vi "ShooterSpeed.vi"(8 "semaphore":T1, 9 "Bottom Shooter":T2, 10 "Top Shooter":T2) -> ()   [LabVIEW 2011]
uses:
  <vilib>/Rock Robotics/WPI/MotorControl/WPI_MotorControlDeviceRef.ctl
  <vilib>/Rock Robotics/SystemInterfaces/Typedef/FPGA_TypedefDigitalModule.ctl
  <vilib>/Rock Robotics/SystemInterfaces/DIO/FPGA_DIOPWMChannel.ctl
  <vilib>/Rock Robotics/WPI/PWM/WPI_PWMDeadband.ctl
  <vilib>/Rock Robotics/WPI/CAN/Jaguar/SubVIs/WPI_CANJaguar_ControlMode.ctl
  <vilib>/Rock Robotics/WPI/PWM/WPI_PWMTransform_ConPane.ctl
  Robot Global Data.vi
  <vilib>/addons/control/pid/NI_PID_pid.lvlib
panel:
  in  "t":dbl
  out "PID Out":dbl(graph)
  out "Error":dbl(graph)
  in  "Shooter Feed Forward":cluster{"Speed":sgl, "Setpoint":sgl}[](array[cluster])=[{"Speed"=0.0, "Setpoint"=0.0}, {"Speed"=1700.0, "Setpoint"=0.3}, {"Speed"=2300.0, "Setpoint"=0.4}, {"Speed"=3000.0, "Setpoint"=0.5}, {"Speed"=3600.0, "Setpoint"=0.6}, {"Speed"=4200.0, "Setpoint"=0.7}, {"Speed"=5000.0, "Setpoint"=0.8}, {"Speed"=6000.0, "Setpoint"=0.9}, {"Speed"=6400.0, "Setpoint"=1.0}]
  out "error out 2":errorcluster
  out "error out":errorcluster
  out "RPM":dbl(graph)
  in  "PID gains":T8={"proportional gain (Kc)"=8.0, "integral time (Ti, min)"=0.01, "derivative time (Td, min)"=0.0} {"derivative time (Td, min)" format="%.3f"; "integral time (Ti, min)" format="%.3f"; "proportional gain (Kc)" format="%.3f"}
  in  "output range":cluster{"output high":dbl, "output low":dbl}={"output high"=0.5, "output low"=-0.5} {"output low" format="%.2f"; "output high" format="%.2f"}
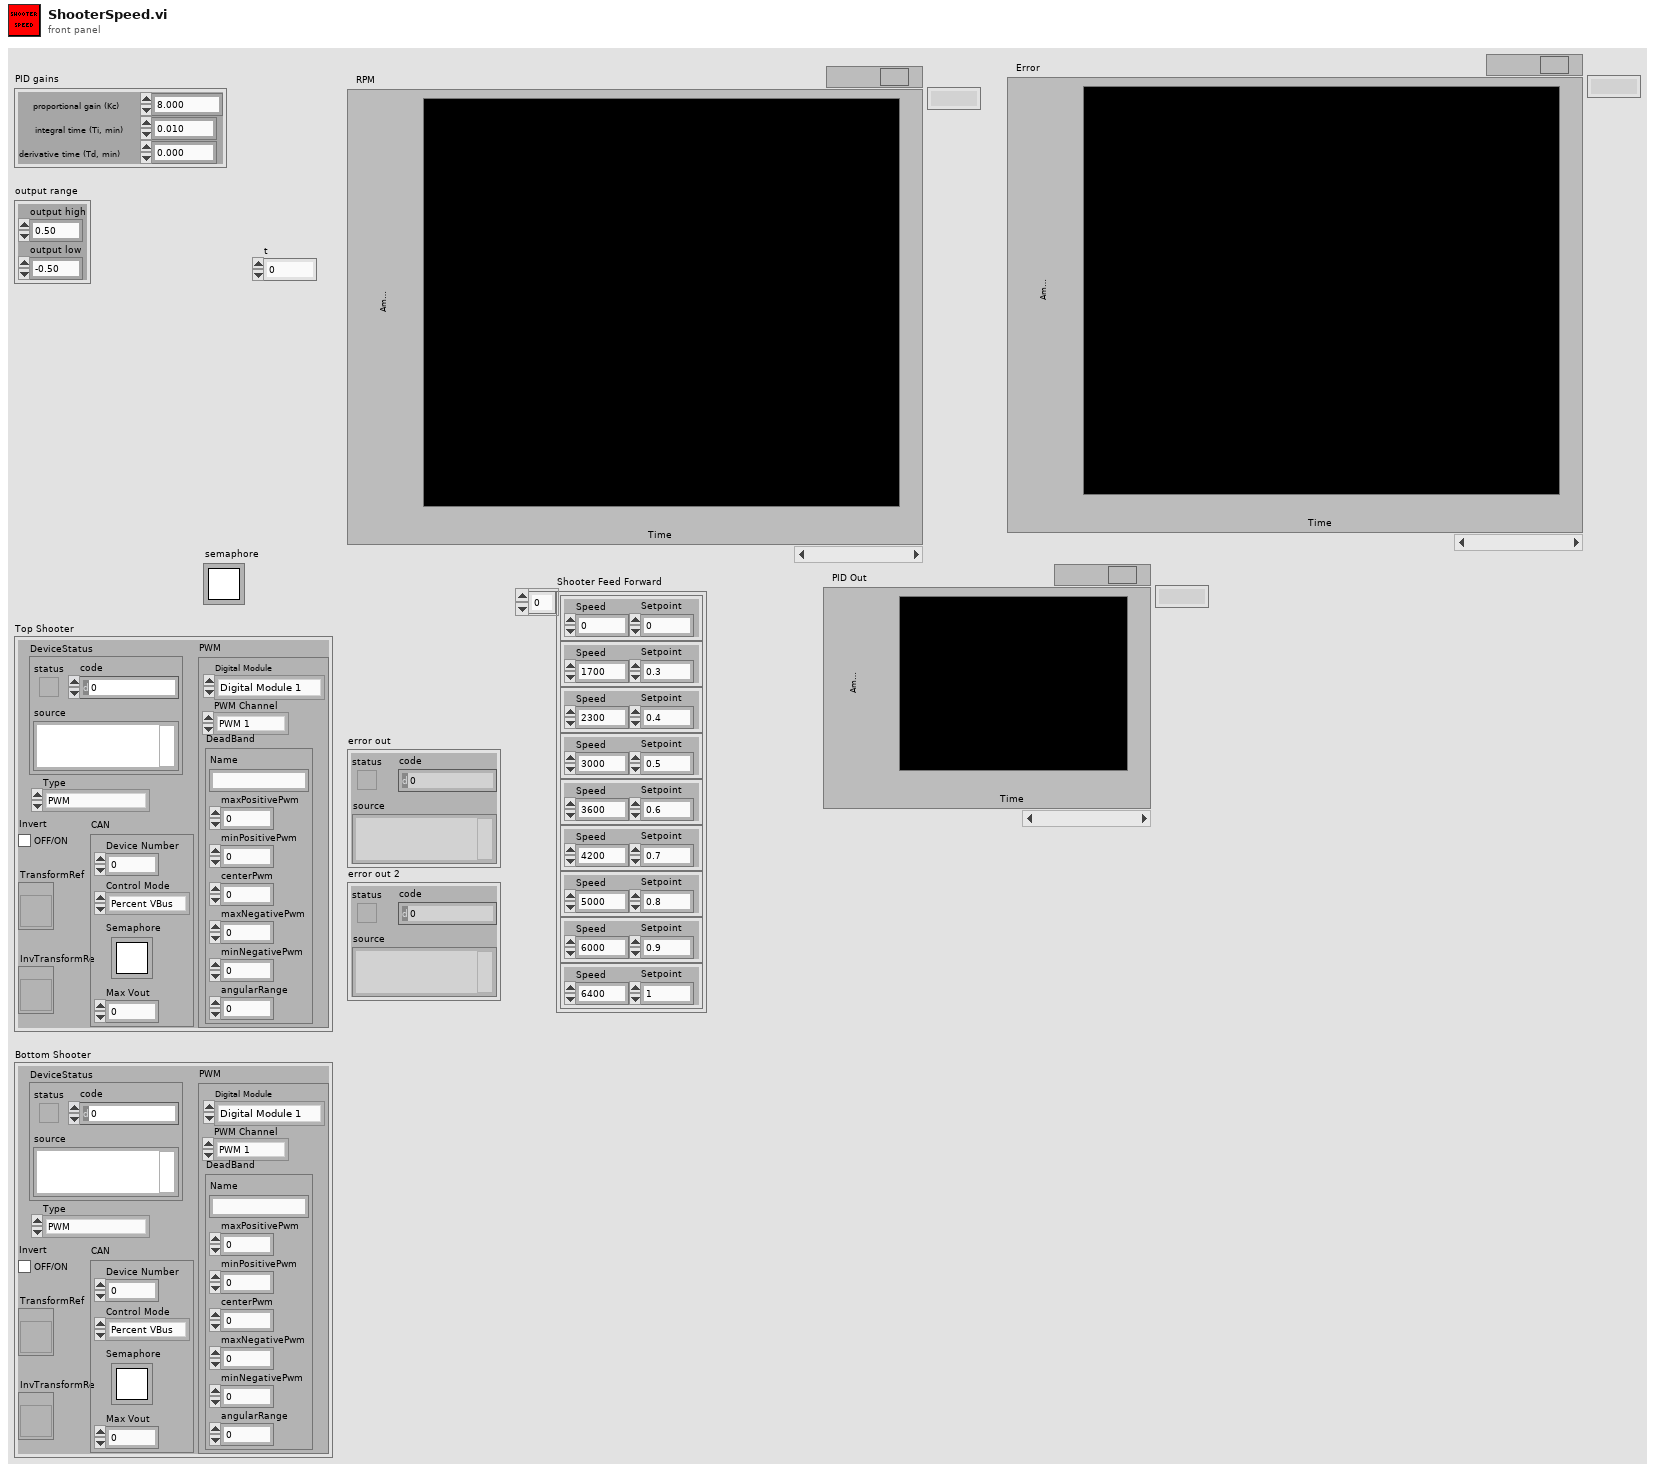
[diagram p1: front panel]
types:
  T1 = typedef "Semaphore RefNum" = refnum<k1>
  T2 = typedef "WPI_MotorControlDeviceRef.ctl" = cluster{"DeviceStatus":errorcluster, "Type":enum16{"PWM", "CAN"}, "PWM":cluster{"Digital Module":T3, "PWM Channel":T4, "DeadBand":T5}, "CAN":cluster{"Device Number":u8, "Control Mode":T6, "Semaphore":T1, "Max Vout":dbl}, "Invert":bool, "TransformRef":T7, "InvTransformRef":T7}
  T3 = typedef "FPGA_TypedefDigitalModule.ctl" = enum16{"Digital Module 1", "Digital Module 2"}
  T4 = typedef "FPGA_DIOPWMChannel.ctl" = enum8{"PWM 1", "PWM 2", "PWM 3", "PWM 4", "PWM 5", "PWM 6", "PWM 7", "PWM 8", "PWM 9", "PWM 10", "Invalid"}
  T5 = typedef "WPI_PWMDeadband.ctl" = cluster{"Name":string, "maxPositivePwm":i32, "minPositivePwm":i32, "centerPwm":i32, "maxNegativePwm":i32, "minNegativePwm":i32, "angularRange":u16}
  T6 = typedef "WPI_CANJaguar_ControlMode.ctl" = enum8{"Percent VBus", "Current", "Speed", "Position", "Voltage"}
  T7 = typedef "WPI_PWMTransform_ConPane.ctl" = refnum<vi>
  T8 = cluster{"proportional gain (Kc)":dbl, "integral time (Ti, min)":dbl, "derivative time (Td, min)":dbl}
  T9 = typedef "ShooterData.ctl" = cluster{"Setpoint":dbl, "Speed":dbl, "Squish":dbl, "Shot Sensor":bool, "At Speed":bool}
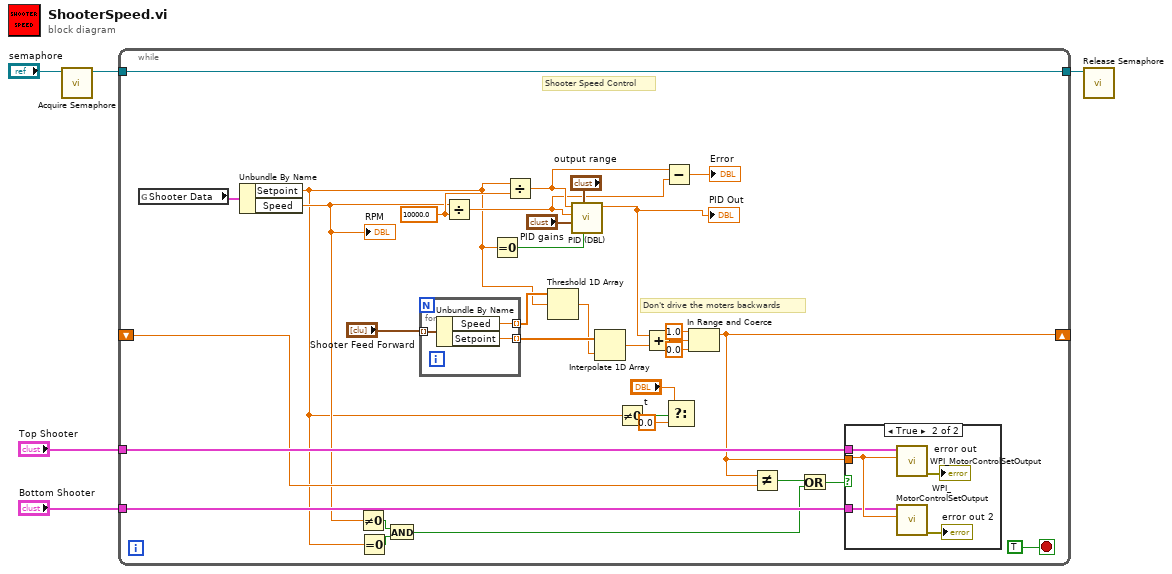
[diagram p0: block diagram]
diagram:
  n1 = call <vilib>:"Acquire Semaphore.vi"("semaphore"="semaphore") -> ("semaphore out"=w3:T1)  [unwired: 4 in, 2 out]
  n2 = while {
    tunnel: "Top Shooter" -> [w37]
    tunnel: "Bottom Shooter" -> [w36]
    tunnel: w3 -> [w34]
    tunnel: [w34] -> w2
    shift-right: [w6] -> _
    shift-left: _ -> [w21]
    stop <- TRUE stop-if-true
    w30 = 10000.0 ("y")
    # "Don't drive the moters backwards"
    # "Shooter Speed Control"
    n3 = global read "Robot Global Data.vi" "Shooter Data"() -> (w35:T9)
    n4 = Unbundle By Name(w35) -> ("Setpoint"=w9:dbl, "Speed"=w16:dbl)
    "RPM" <- w16
    n5 = Not Equal To 0?(x=w16) -> (x != 0?=w17:bool)
    n6 = Equal To 0?(x=w9) -> (x = 0?=w18:bool)
    n7 = And(x=w17, y=w18) -> (x .and. y?=w15:bool)
    n8 = for {
      tunnel: "Shooter Feed Forward" -> [w41] mode=indexing
      tunnel: [w40] -> w27 mode=indexing
      tunnel: [w39] -> w29 mode=indexing
      n9 = Unbundle By Name(w41) -> ("Speed"=w40:sgl, "Setpoint"=w39:sgl)
    }
    n10 = Divide(x=w16, y=w30) -> (x/y=w13:dbl)
    n11 = Equal To 0?(x=w9) -> (x = 0?=w33:bool)
    n12 = Divide(x=w9, y=w30) -> (x/y=w14:dbl)
    n13 = Threshold 1D Array(2:w9, 3:w27) -> (0:w28:sgl)  [unwired: 1 in]
    n14 = call <vilib>:"PID (DBL).vi"("reinitialize? (F)"=w33, "output range"="output range", "PID gains"="PID gains", "process variable"=w13, "setpoint"=w14) -> ("output"=w12:dbl)  [unwired: 1 in, 5 out]
    "PID Out" <- w12
    n15 = Interpolate 1D Array(1:w28, 2:w29) -> (0:w25:sgl)
    n16 = Not Equal To 0?(x=w9) -> (x != 0?=w10:bool)
    n17 = Add(x=w12, y=w25) -> (x+y=w24:dbl)
    n18 = Subtract(x=w14, y=w13) -> (x-y=→"Error":dbl)
    n19 = Select(t="t", s=w10, f=0.0) -> ()  [unwired: 1 out]
    n20 = In Range and Coerce(upper limit=1.0, x=w24, lower limit=0.0) -> (coerced(x)=w6:dbl)  [unwired: 1 out]
    n21 = Not Equal?(x=w6, y=w21) -> (x != y?=w19:bool)
    n22 = Or(x=w19, y=w15) -> (x .or. y?=w20:bool)
    n23 = case shown="True" w20 {
      tunnel: w6 -> [_ w46]
      tunnel: w37 -> [_ w45]
      tunnel: w36 -> [_ w44]
      frame False {
      }
      frame True {
        n24 = call <vilib>:"WPI_MotorControlSetOutput.vi"("Output"=w46, "MotorControlDevRef"=w45) -> ("error out"=→"error out":errorcluster)  [unwired: 8 in, 1 out]
        n25 = call <vilib>:"WPI_MotorControlSetOutput.vi"("Output"=w46, "MotorControlDevRef"=w44) -> ("error out"=→"error out 2":errorcluster)  [unwired: 8 in, 1 out]
      }
    }
  }
  n26 = call <vilib>:"Release Semaphore.vi"("semaphore"=w2) -> ()  [unwired: 5 in, 2 out]
